vi "Initialize With Dialog.vi"(8 "error in (no error)":errorcluster, 11 "Sound Player in":refnum<class "Sound Player.lvclass">) -> (0 "error out":errorcluster, 2 "Cancelled?":bool, 3 "Sound Player out":refnum<class "Sound Player.lvclass">)   [LabVIEW 2017, in "Sound Player.lvclass"]
doc: "Launch a dialog that allows configuration of the sound player. The Sound Player class itself has no configuration, but this VI is fully written as a dialog VI so it can be used as an easier starting template for child classes than the regular Dialog With Events template that ships with LV because this one already has the input/output terminals needed for the dynamic dispatching and error handling. Child classes that truly have no configuration needs should override this VI with a VI that does nothing but return the unmodified input object. \n\nThis VI is marked as Must Override."
uses:
  Sound Player.lvclass
panel:
  in  "Cancel":bool
  in  "OK":bool
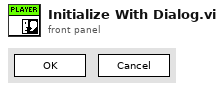
[diagram p1: front panel]
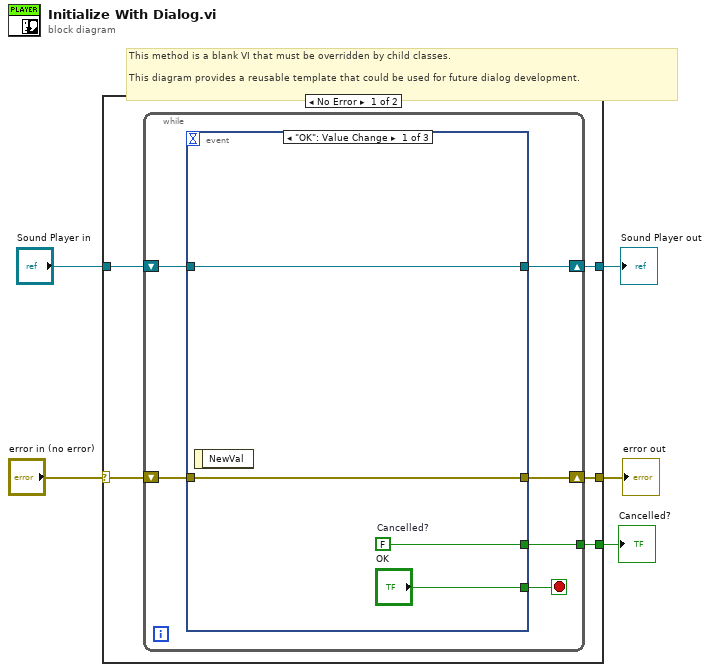
[diagram p0: block diagram]
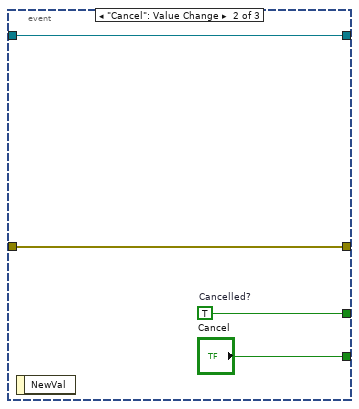
[diagram p2: hidden frame]
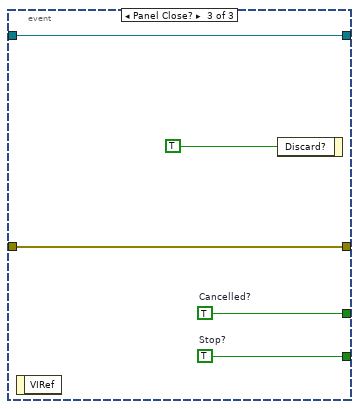
[diagram p3: hidden frame]
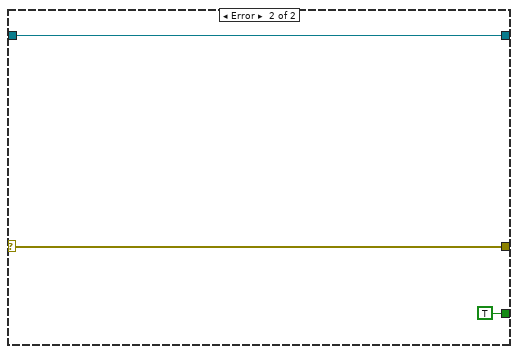
[diagram p4: hidden frame]
diagram:
  # "This method is a blank VI that must be overridden by child classes.  \n\nThis diagram provides a reusable template that could be used for future dialog development."
  n1 = case shown="No Error" "error in (no error)" {
    selector: "error in (no error)" -> [w8 w32]
    tunnel: [w10 TRUE ("Cancelled?")] -> w5
    tunnel: [w7 w32] -> w3
    tunnel: [w9 w31] -> w2
    tunnel: "Sound Player in" -> [w6 w31]
    frame No Error {
      n2 = while {
        tunnel: [w15] -> w10
        shift-right: [w14] -> w9
        shift-left: w6 -> [w13]
        shift-right: [w11] -> w7
        shift-left: w8 -> [w12]
        stop <- w16 stop-if-true
        n3 = event shown="[0] \"OK\": Value Change" {
          selector: _ -> [_ _ _]
          dyn-events: _ -> [_ _ _]
          timeout: _ -> [_ _ _]
          tunnel: ["OK" "Cancel" w28] -> w16
          tunnel: [w20 w24 w27] -> w15
          tunnel: [w18 w22 w26] -> w14
          tunnel: w13 -> [w18 w22 w26]
          tunnel: w12 -> [w17 w21 w25]
          tunnel: [w17 w21 w25] -> w11
          event "OK": Value Change {
            w20 = FALSE  # Cancelled?
            n4 = event-data() -> ()  [unwired: 1 in, 1 out]
          }
          event "Cancel": Value Change {
            w24 = TRUE  # Cancelled?
            n5 = event-data() -> ()  [unwired: 1 in, 1 out]
          }
          event Panel Close? {
            w27 = TRUE  # Cancelled?
            w28 = TRUE  # Stop?
            n6 = event-data() -> ()  [unwired: 1 in, 1 out]
            n7 = event-data("Discard?"=TRUE) -> ()  [unwired: 1 in, 1 out]
          }
        }
      }
    }
    frame Error {
    }
  }
  "Cancelled?" <- w5
  "Sound Player out" <- w2
  "error out" <- w3
